vi "Display Running.vi"() -> ()   [LabVIEW 2017]
panel:
  out "Numeric":i32
  out "Slide":u8(slide) scale=0.0..100.0
  # "%"
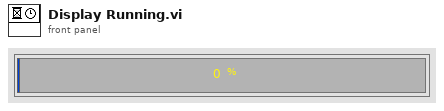
[diagram p1: front panel]
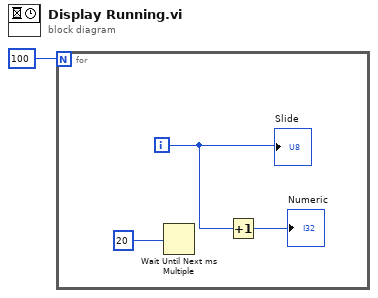
[diagram p0: block diagram]
diagram:
  n1 = for {
    N: 100 -> [_]
    i -> [w3]
    n2 = Wait Until Next ms Multiple(millisecond multiple=20) -> ()  [unwired: 1 out]
    n3 = Increment(x=w3) -> (x+1=→"Numeric":i32)
    "Slide" <- w3
  }
